vi "Read Page.vi"(8 "error in (no error)":errorcluster, 10 "index":i32, 11 "TIFF Reader in":refnum<class "TIFF Reader.lvclass">) -> (0 "error out":errorcluster, 1 "Details":T3={"ImageDescription"="", "XResolution"=0.0, "YResolution"=0.0, "ResolutionUnit"=enum."Inch", "PhotometricInterpretation"=0, "Compression"=enum."None", "PageName"="", "DocumentName"=""} {"PhotometricInterpretation" items=["MIN IS WHITE"=0, "MIN IS BLACK"=1, "RGB"=2, "PALETTE"=3, "MASK"=4, "SEPARATED"=5, "YCBCR"=6, "CIE LAB"=8, "ICC LAB"=9, "ITU LAB"=10, "LOGL"=32844, "LOGLUV"=32845, "CFA"=32803, "LinearRaw"=34892, "DEPTH"=51177]}, 2 "Image Data":variant, 3 "TIFF Reader out":refnum<class "TIFF Reader.lvclass">, 4 "IFD Info":T2(c390))   [LabVIEW 2020, in "LV Tiff.lvlib" / "TIFF Reader.lvclass"]
uses:
  TIFF Reader.lvclass
  _Helpers/Tiff Page Details.ctl
  _Helpers/Tiff Data Type.ctl
  TIFF Reader.lvclass/TIFF Reader.ctl
  LV Tiff.lvlib
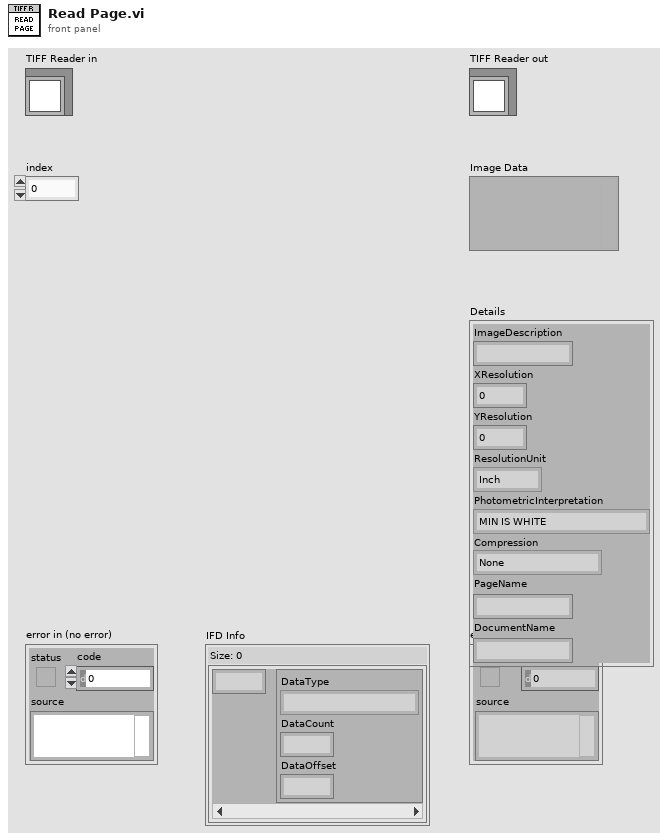
[diagram p1: front panel]
types:
  T1 = typedef "LV Tiff.lvlib/Tiff Data Type.ctl" = enum16{"Null", "BYTE", "ASCII", "SHORT", "LONG", "RATIONAL", "SBYTE", "UNDEFINE", "SSHORT", "SLONG", "SRATIONAL", "FLOAT", "DOUBLE"}
  T2 = map{u16, cluster{"DataType":T1, "DataCount":u32, "DataOffset":u32}}
  T3 = typedef "LV Tiff.lvlib/Tiff Page Details.ctl" = cluster{"ImageDescription":string, "XResolution":dbl, "YResolution":dbl, "ResolutionUnit":enum16{"None", "Inch", "Centimeter"}, "PhotometricInterpretation":u16, "Compression":enum16{"None", "Deflate"}, "PageName":string, "DocumentName":string}
  T4 = enum16{"big-endian, network order", "native, host order", "little-endian"}
  T5 = cluster{i32, "Array":cluster{"TagID":u16, "DataType":T1, "DataCount":u32, "DataOffset":u32}[], "IFDOffset":u32}[]
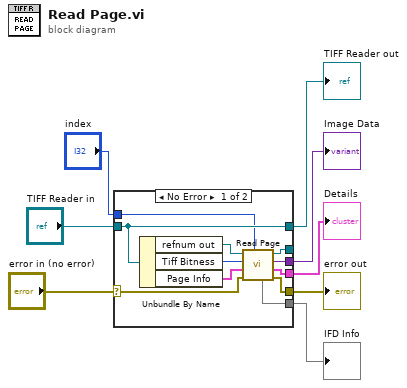
[diagram p0: block diagram]
diagram:
  n1 = case shown="No Error" "error in (no error)" {
    selector: "error in (no error)" -> [w19 w21]
    tunnel: [w18 w21] -> w7
    tunnel: [w17 w20] -> w5
    tunnel: "TIFF Reader in" -> [w17 w20]
    tunnel: "index" -> [w13 _]
    tunnel: [w12 _] -> _
    tunnel: [w11 _] -> w3
    tunnel: [w10 _] -> w2
    tunnel: [w9 _] -> w1
    frame No Error {
      n2 = Unbundle By Name(w17) -> ("refnum out"=w16:refnum<file>, "Tiff Bitness"=w15:T4, "Page Info"=w14:T5)
      n3 = call "Read Page.vi"("index"=w13, "error in (no error)"=w19, "Page Info"=w14, "Tiff Bitness"=w15, "Byte Stream File in"=w16) -> ("error out"=w18:errorcluster, "Details"=w10:T3, "Variant"=w11:variant, "Byte Stream File out"=w12:refnum<file>, "IFD Info"=w9:T2)  [unwired: 2 in]
    }
    frame Error {
    }
  }
  "error out" <- w7
  "TIFF Reader out" <- w5
  "Image Data" <- w3
  "Details" <- w2
  "IFD Info" <- w1
